vi "Calculate_Angles_for_Subtracks_(101-11)-1.vi"(5 "[IN] Index of subtrack":i32, 6 "[IN] Subtrack":dbl[](array[numeric]), 7 "[IN] Index of \"101\" Dis-\nplacement in Subtrack":i32, 8 "[IN] Reverse Displ or Not":bool[](array[boolean]), 9 "[IN] Array with Angles \nBetween Displacement":dbl[](array[numeric])) -> (2 "[OUT] Reverse displacement or not":bool[](array[boolean]), 3 "[OUT] Angles betwe\nen two displacements":dbl[](array[numeric]))   [LabVIEW 2013]
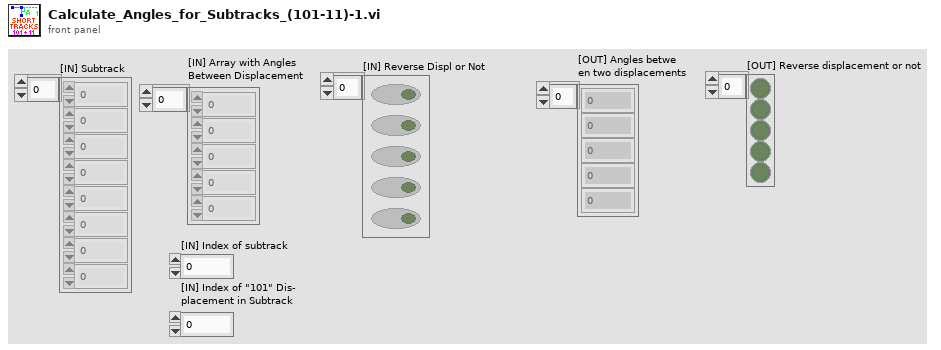
[diagram p1: front panel]
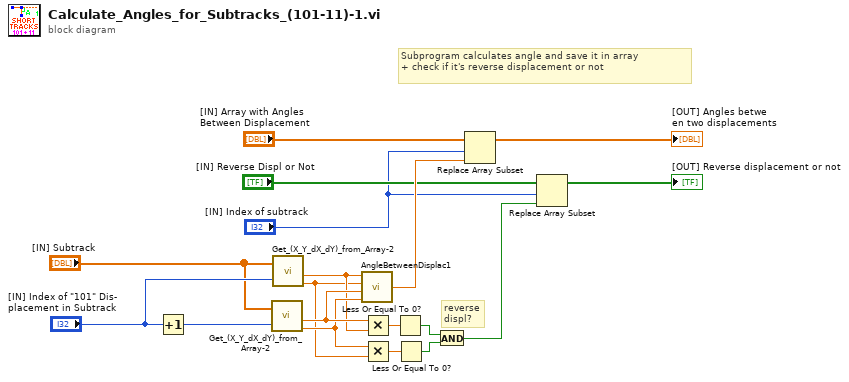
[diagram p0: block diagram]
diagram:
  # "Subprogram calculates angle and save it in array \n+ check if it's reverse displacement or not"
  # "reverse \ndispl?"
  n1 = Increment(x="[IN] Index of \"101\" Dis-\nplacement in Subtrack") -> (x+1=w1:i32)
  n2 = call "Get_(X_Y_dX_dY)_from_Array-2.vi"("(X,Y,dX,dY)"="[IN] Subtrack", "Index of Displacement"=w1) -> ("dX"=w12:dbl, "dY"=w11:dbl)  [unwired: 2 out]
  n3 = call "Get_(X_Y_dX_dY)_from_Array-2.vi"("(X,Y,dX,dY)"="[IN] Subtrack", "Index of Displacement"="[IN] Index of \"101\" Dis-\nplacement in Subtrack") -> ("dX"=w10:dbl, "dY"=w9:dbl)  [unwired: 2 out]
  n4 = call "AngleBetweenDisplac1.vi"("dY 2"=w11, "dX 2"=w12, "dY 1"=w9, "dX 1"=w10) -> ("angle in degrees"=w7:dbl)
  n5 = Multiply(x=w12, y=w10) -> (x*y=w16:dbl)
  n6 = Multiply(x=w11, y=w9) -> (x*y=w15:dbl)
  n7 = Less Or Equal To 0?(x=w16) -> (x <= 0?=w13:bool)
  n8 = Less Or Equal To 0?(x=w15) -> (x <= 0?=w14:bool)
  n9 = And(x=w13, y=w14) -> (x .and. y?=w4:bool)
  n10 = Replace Array Subset(array="[IN] Array with Angles \nBetween Displacement", new element=w7, index="[IN] Index of subtrack") -> (→"[OUT] Angles betwe\nen two displacements":dbl[])
  n11 = Replace Array Subset(array="[IN] Reverse Displ or Not", new element=w4, index="[IN] Index of subtrack") -> (→"[OUT] Reverse displacement or not":bool[])
